vi "Read Attributes.vi"(11 "Tx Root Content Msg":refnum<class "Tx Root Content Msg.lvclass">) -> (2 "Payload":cluster{"Content":string})   [LabVIEW 2020, in "Nested Actor.lvlib" / "Tx Root Content Msg.lvclass"]
uses:
  Tx Root Content Msg.lvclass
  Tx Root Content Msg.lvclass/Tx Root Content Msg.ctl
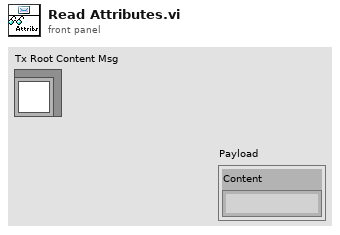
[diagram p1: front panel]
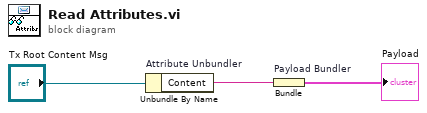
[diagram p0: block diagram]
diagram:
  n1 = Unbundle By Name "Attribute Unbundler"("Tx Root Content Msg") -> ("Content"=w1:string)
  n2 = Bundle "Payload Bundler"("Content"=w1) -> (→"Payload":cluster{"Content":string})  [unwired: 1 in]
